vi "GetAgregateAlarm.vi"(0 "reference in":refnum<class "AI.lvclass">, 11 "error in (no error)":errorcluster) -> (4 "reference out":refnum<class "AI.lvclass">, 6 "Alarm":bool, 8 "Warning":bool, 15 "error out":errorcluster)   [LabVIEW 2019, in "AI.lvclass"]
uses:
  AI.lvclass
  AI.lvclass/AI.ctl
  AnalogComparator_class/AnalogComparator.lvclass/AnalogComparator.ctl
  AnalogComparator_class/AnalogComparator.lvclass
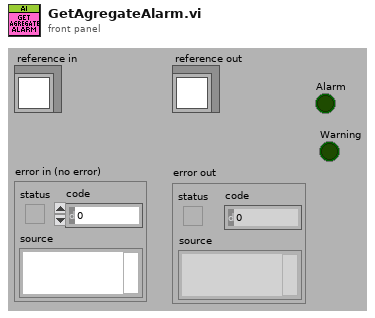
[diagram p1: front panel]
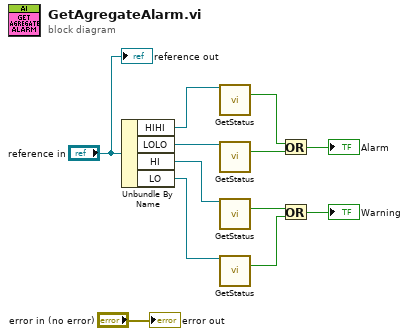
[diagram p0: block diagram]
diagram:
  n1 = Unbundle By Name("reference in") -> ("HIHI"=w9:refnum<class "AnalogComparator.lvclass">, "LOLO"=w7:refnum<class "AnalogComparator.lvclass">, "HI"=w2:refnum<class "AnalogComparator.lvclass">, "LO"=w1:refnum<class "AnalogComparator.lvclass">)
  n2 = call "GetStatus.vi"("class data in"=w9) -> ("Status"=w8:bool)  [unwired: 14 in]
  n3 = call "GetStatus.vi"("class data in"=w7) -> ("Status"=w6:bool)  [unwired: 14 in]
  n4 = call "GetStatus.vi"("class data in"=w2) -> ("Status"=w4:bool)  [unwired: 14 in]
  n5 = call "GetStatus.vi"("class data in"=w1) -> ("Status"=w5:bool)  [unwired: 14 in]
  n6 = Or(x=w8, y=w6) -> (x .or. y?=→"Alarm":bool)
  n7 = Or(x=w4, y=w5) -> (x .or. y?=→"Warning":bool)
  "error out" <- "error in (no error)"
  "reference out" <- "reference in"
